vi "MOTOR SIMULADO.vi"(11 "Voltaje":dbl(slide) scale=-100.0..100.0) -> (3 "Posicion":dbl(knob))   [LabVIEW 2013]
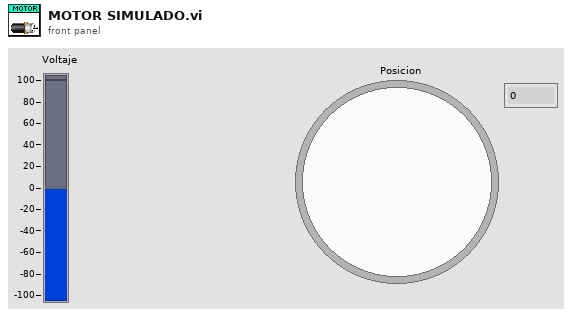
[diagram p1: front panel]
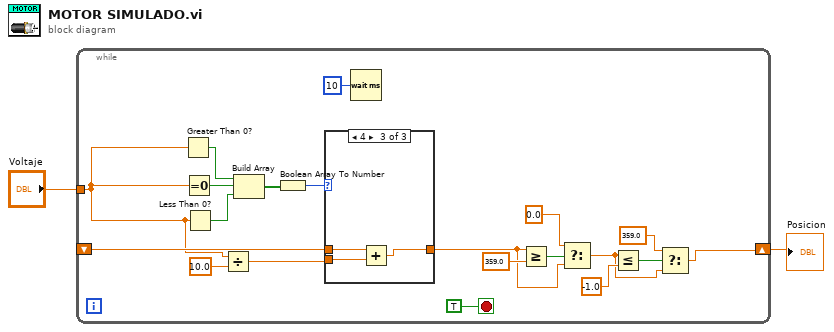
[diagram p0: block diagram]
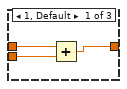
[diagram p2: hidden frame]
diagram:
  n1 = while {
    shift-right: [w7] -> w1
    shift-left: _ -> [w16]
    tunnel: "Voltaje" -> [w3]
    stop <- TRUE stop-if-true
    n2 = Greater Than 0?(x=w3) -> (x > 0?=w20:bool)
    n3 = Equal To 0?(x=w3) -> (x = 0?=w21:bool)
    n4 = Less Than 0?(x=w3) -> (x < 0?=w19:bool)
    n5 = Divide(x=w3, y=10.0) -> (x/y=w5:dbl)
    n6 = Build Array(w20, w21, w19) -> (w18:bool[])
    n7 = Boolean Array To Number(Boolean array=w18) -> (number=w17:u32)
    n8 = case shown="4" w17 {
      tunnel: w16 -> [w25 w26 w29]
      tunnel: [w23 w26 w27] -> w12
      tunnel: w5 -> [w24 _ w28]
      frame 1, Default {
        n9 = Add(x=w25, y=w24) -> (x+y=w23:dbl)
      }
      frame 2 {
      }
      frame 4 {
        n10 = Add(x=w29, y=w28) -> (x+y=w27:dbl)
      }
    }
    n11 = Wait (ms)(milliseconds to wait=u32 10) -> ()  [unwired: 1 out]
    n12 = Greater Or Equal?(x=w12, y=359.0) -> (x >= y?=w14:bool)
    n13 = Select(t=0.0, s=w14, f=w12) -> (s? t:f=w8:dbl)
    n14 = Less Or Equal?(x=w8, y=-1.0) -> (x <= y?=w10:bool)
    n15 = Select(t=359.0, s=w10, f=w8) -> (s? t:f=w7:dbl)
  }
  "Posicion" <- w1
